vi "RUSHShoot.vi"(1 "In Cluster":T3={"ShootTrackEnable"=FALSE, "ShootStartWheels"=FALSE, "ShootIndexerEnable"=FALSE, "ShootCase"=0.0, "ShootPOTElev"=0.0, "ShootManualElev"=0.0, "IndexerSpeed"=0.0, "Wheel Spd F"=0.0, "Deadband"=0.0, "ShootTargetInfo"={"X Coord"=0.0, "Y Coord"=0.0, "Distance"=0.0}, "ShootConstElev"={"1"=0.0, "2"=0.0, "3"=0.0, "4"=0.0, "Ground"=0.0}, "ShootRollerSpd"=0.0, "ShootFlipperPE"=FALSE, "Wheel Spd B"=0.0, "ShootConstFlipper"={"Down 1"=0.2, "Up 1"=0.8, "Up 2"=0.8, "Down 2"=0.2}}) -> (0 "Out Cluster":T2)   [LabVIEW 2012]
uses:
  <vilib>/Rock Robotics/WPI/Relay/WPI_RelayValue.ctl
panel:
  in  "Highest POT pos":dbl=4.2
  in  "Lowest POT pos":dbl=2.1
  in  "ShootPOTToPowConst":dbl=1.0
  in  "Vision Speed Const":dbl=0.75
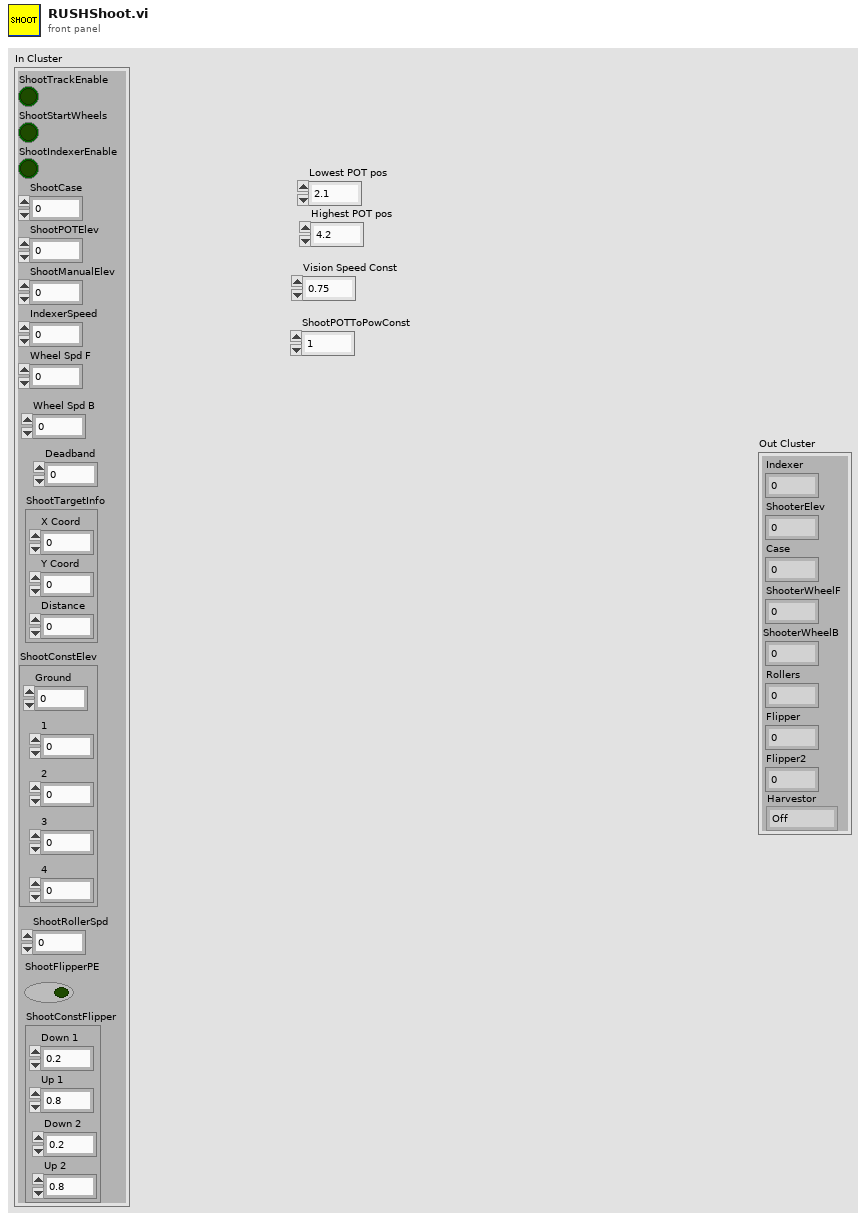
[diagram p1: front panel]
types:
  T1 = typedef "WPI_RelayValue.ctl" = enum16{"Off", "On", "Forward", "Reverse"}
  T2 = cluster{"Indexer":dbl, "ShooterElev":dbl, "Case":dbl, "ShooterWheelF":dbl, "ShooterWheelB":dbl, "Rollers":dbl, "Flipper":dbl, "Flipper2":dbl, "Harvestor":T1}
  T3 = cluster{"ShootTrackEnable":bool, "ShootStartWheels":bool, "ShootIndexerEnable":bool, "ShootCase":dbl, "ShootPOTElev":dbl, "ShootManualElev":dbl, "IndexerSpeed":dbl, "Wheel Spd F":dbl, "Deadband":dbl, "ShootTargetInfo":cluster{"X Coord":dbl, "Y Coord":dbl, "Distance":dbl}, "ShootConstElev":cluster{"1":dbl, "2":dbl, "3":dbl, "4":dbl, "Ground":dbl}, "ShootRollerSpd":dbl, "ShootFlipperPE":bool, "Wheel Spd B":dbl, "ShootConstFlipper":cluster{"Down 1":dbl, "Up 1":dbl, "Up 2":dbl, "Down 2":dbl}}
  T4 = cluster{"X Coord":dbl, "Y Coord":dbl, "Distance":dbl}
  T5 = cluster{"1":dbl, "2":dbl, "3":dbl, "4":dbl, "Ground":dbl}
  T6 = cluster{"Down 1":dbl, "Up 1":dbl, "Up 2":dbl, "Down 2":dbl}
  T7 = cluster{"f":dbl, "y":dbl, "f":dbl, "f":dbl, "f":dbl, "f":dbl, "Down 1":dbl, "Down 2":dbl, "Harvestor":T1}
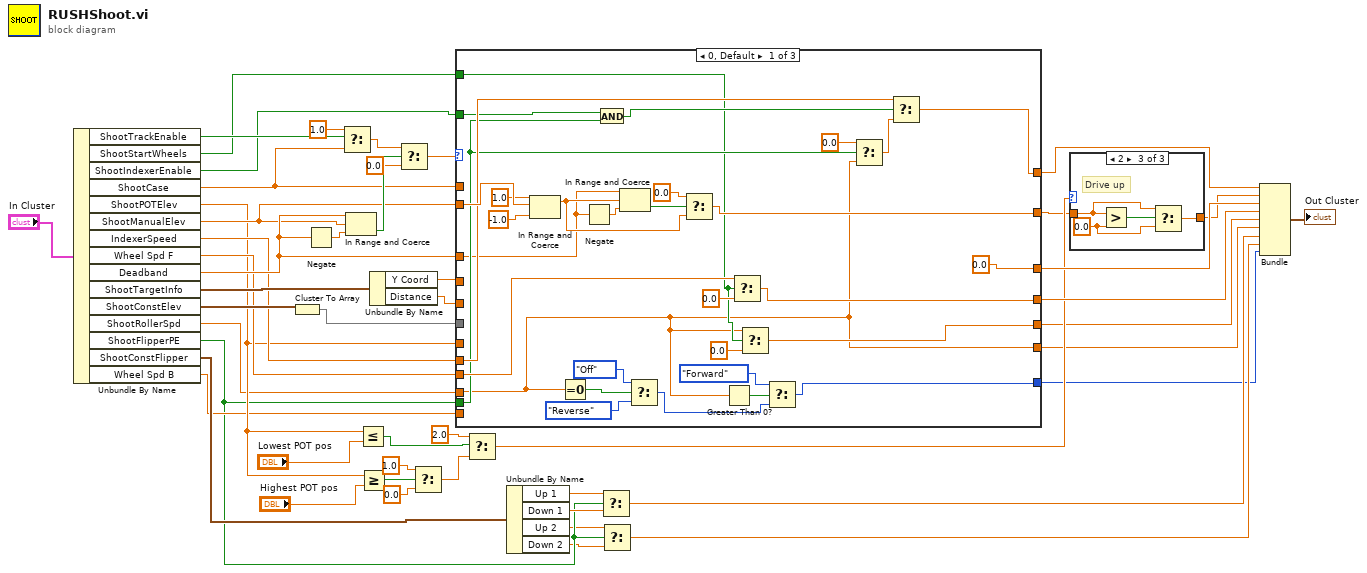
[diagram p0: block diagram]
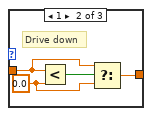
[diagram p3: hidden frame]
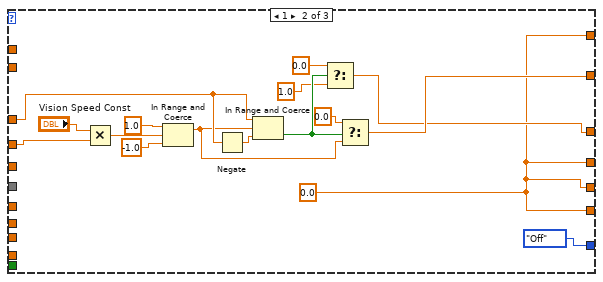
[diagram p4: hidden frame]
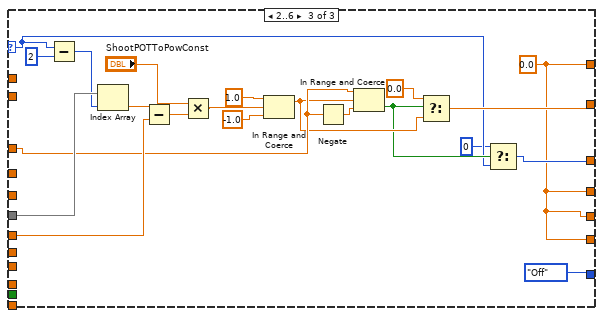
[diagram p5: hidden frame]
diagram:
  n1 = Unbundle By Name("In Cluster") -> ("ShootTrackEnable"=w48:bool, "ShootStartWheels"=w36:bool, "ShootIndexerEnable"=w35:bool, "ShootCase"=w37:dbl, "ShootPOTElev"=w25:dbl, "ShootManualElev"=w34:dbl, "IndexerSpeed"=w28:dbl, "Wheel Spd F"=w27:dbl, "Deadband"=w38:dbl, "ShootTargetInfo"=w41:T4, "ShootConstElev"=w33:T5, "ShootRollerSpd"=w14:dbl, "ShootFlipperPE"=w6:bool, "ShootConstFlipper"=w12:T6, "Wheel Spd B"=w10:dbl)
  n2 = Cluster To Array(cluster=w33) -> (array=w32:dbl[])
  n3 = Negate(x=w38) -> (-x=w45:dbl)
  n4 = Select(t=1.0, s=w48, f=w37) -> (s? t:f=w46:dbl)
  n5 = In Range and Coerce(upper limit=w38, x=w34, lower limit=w45) -> (In Range?=w44:bool)  [unwired: 1 out]
  n6 = Less Or Equal?(x=w25, y="Lowest POT pos") -> (x <= y?=w19:bool)
  n7 = Greater Or Equal?(x=w25, y="Highest POT pos") -> (x >= y?=w23:bool)
  n8 = Unbundle By Name(w41) -> ("Y Coord"=w40:dbl, "Distance"=w39:dbl)
  n9 = Select(t=w46, s=w44, f=0.0) -> (s? t:f=w42:dbl)
  n10 = Select(t=1.0, s=w23, f=0.0) -> (s? t:f=w20:dbl)
  n11 = case shown="0, Default" w42 {
    selector: w42 -> [_ _ w101]
    tunnel: w40 -> [_ w95 _]
    tunnel: w39 -> [_ _ _]
    tunnel: w38 -> [w61 w90 w106]
    tunnel: [0.0 ("upper limit") w84 w99] -> w30
    tunnel: w37 -> [_ _ _]
    tunnel: [w73 w85 w103] -> w16
    tunnel: [w71 w82 w98] -> w29
    tunnel: [w80 w82 w98] -> w31
    tunnel: w36 -> [w59 _ _]
    tunnel: w35 -> [w66 _ _]
    tunnel: w34 -> [w77 _ _]
    tunnel: w32 -> [_ _ w116]
    tunnel: w25 -> [_ _ w113]
    tunnel: w28 -> [w67 _ _]
    tunnel: w27 -> [w68 _ _]
    tunnel: w14 -> [w50 _ _]
    tunnel: [w50 w82 w98] -> w8
    tunnel: w6 -> [w64 _ _]
    tunnel: w10 -> [_ _ _]
    tunnel: [w58 w82 w98] -> w7
    tunnel: [w51 WPI_RelayValue."Off" ("Harvestor") WPI_RelayValue."Off" ("Harvestor")] -> w2
    frame 0, Default {
      n12 = In Range and Coerce(upper limit=1.0, x=w77, lower limit=-1.0 ("upper limit")) -> (coerced(x)=w74:dbl)  [unwired: 1 out]
      n13 = Equal To 0?(x=w50) -> (x = 0?=w55:bool)
      n14 = Negate(x=w61) -> (-x=w78:dbl)
      n15 = And(x=w66, y=w64) -> (x .and. y?=w65:bool)
      n16 = In Range and Coerce(upper limit=w61, x=w74, lower limit=w78) -> (In Range?=w76:bool)  [unwired: 1 out]
      n17 = Select(t=WPI_RelayValue."Off" ("Harvestor"), s=w55, f=WPI_RelayValue."Reverse" ("Harvestor")) -> (s? t:f=w52:T1)
      n18 = Select(t=0.0, s=w76, f=w74) -> (s? t:f=w73:dbl)
      n19 = Greater Than 0?(x=w50) -> (x > 0?=w57:bool)
      n20 = Select(t=w68, s=w59, f=0.0 ("t")) -> (s? t:f=w71:dbl)
      n21 = Select(t=w50, s=w59, f=0.0 ("t")) -> (s? t:f=w58:dbl)
      n22 = Select(t=WPI_RelayValue."Forward" ("Harvestor"), s=w57, f=w52) -> (s? t:f=w51:T1)
      n23 = Select(t=0.0, s=w64, f=w50) -> (s? t:f=w62:dbl)
      n24 = Select(t=w67, s=w65, f=w62) -> (s? t:f=w80:dbl)
    }
    frame 1 {
      w82 = 0.0
      n25 = Multiply(x="Vision Speed Const", y=w95) -> (x*y=w94:dbl)
      n26 = In Range and Coerce(upper limit=1.0, x=w94, lower limit=-1.0 ("upper limit")) -> (coerced(x)=w88:dbl)  [unwired: 1 out]
      n27 = Negate(x=w90) -> (-x=w91:dbl)
      n28 = In Range and Coerce(upper limit=w90, x=w88, lower limit=w91) -> (In Range?=w87:bool)  [unwired: 1 out]
      n29 = Select(t=0.0, s=w87, f=1.0) -> (s? t:f=w84:dbl)
      n30 = Select(t=0.0, s=w87, f=w88) -> (s? t:f=w85:dbl)
    }
    frame 2..6 {
      w98 = 0.0 ("f")
      n31 = Subtract(x=w101, y=2) -> (x-y=w115:i32)
      n32 = Index Array(array=w116, index=w115) -> (element=w114:dbl)
      n33 = Subtract(x=w114, y=w113) -> (x-y=w112:dbl)
      n34 = Multiply(x="ShootPOTToPowConst", y=w112) -> (x*y=w107:dbl)
      n35 = In Range and Coerce(upper limit=1.0, x=w107, lower limit=-1.0 ("upper limit")) -> (coerced(x)=w104:dbl)  [unwired: 1 out]
      n36 = Negate(x=w106) -> (-x=w108:dbl)
      n37 = In Range and Coerce(upper limit=w106, x=w104, lower limit=w108) -> (In Range?=w102:bool)  [unwired: 1 out]
      n38 = Select(t=0.0, s=w102, f=w104) -> (s? t:f=w103:dbl)
      n39 = Select(t=0, s=w102, f=w101) -> (s? t:f=w99:i32)
    }
  }
  n40 = Select(t=2.0, s=w19, f=w20) -> (s? t:f=w17:dbl)
  n41 = Unbundle By Name(w12) -> ("Up 1"=w11:dbl, "Down 1"=w13:dbl, "Up 2"=w5:dbl, "Down 2"=w4:dbl)
  n42 = Select(t=w11, s=w6, f=w13) -> (s? t:f=w9:dbl)
  n43 = Select(t=w5, s=w6, f=w4) -> (s? t:f=w3:dbl)
  n44 = case shown="2" w17 {
    tunnel: w16 -> [w118 w120 w124]
    tunnel: [w118 w119 w123] -> w15
    frame 0, Default {
      # "All good"
    }
    frame 1 {
      w121 = 0.0 ("y")
      # "Drive down"
      n45 = Less?(x=w120, y=w121) -> (x < y?=w122:bool)
      n46 = Select(t=w120, s=w122, f=w121) -> (s? t:f=w119:dbl)
    }
    frame 2 {
      w125 = 0.0 ("y")
      # "Drive up"
      n47 = Greater?(x=w124, y=w125) -> (0:w126:bool)
      n48 = Select(t=w124, s=w126, f=w125) -> (s? t:f=w123:dbl)
    }
  }
  n49 = Bundle("f"=w31, "y"=w15, "f"=w30, "f"=w29, "f"=w7, "f"=w8, "Down 1"=w9, "Down 2"=w3, "Harvestor"=w2) -> (→"Out Cluster":T7)  [unwired: 1 in]
